vi "RTC DS1307 to LCD 16x2.vi"   [LabVIEW 2014]
doc: "This example shows how to read the current time from a DS1307 Real-Time Clock (RTC). This RTC is used on the Arduino Datalogger Shield, which also comes equipped with an SD card slot."
uses:
  <vilib>/Aledyne-TSXperts/Arduino Compatible Compiler for LabVIEW/Code Generator/Arduino APIs/I2C LCD/LiquidCrystal_I2C write String.vi
  <vilib>/Aledyne-TSXperts/Arduino Compatible Compiler for LabVIEW/Arduino Compatible Compiler for LabVIEW.lvlib
  QwaveSys_ESP8266/QwaveSys_ESP8266.lvlib
  QwaveSys_Interface/QwaveSys_Interface.lvlib
panel:
  # "These two wire for I2C (SDA,SCL) must be connected in order to use onboard RTC with Wemos D1 ESP8266 Board"
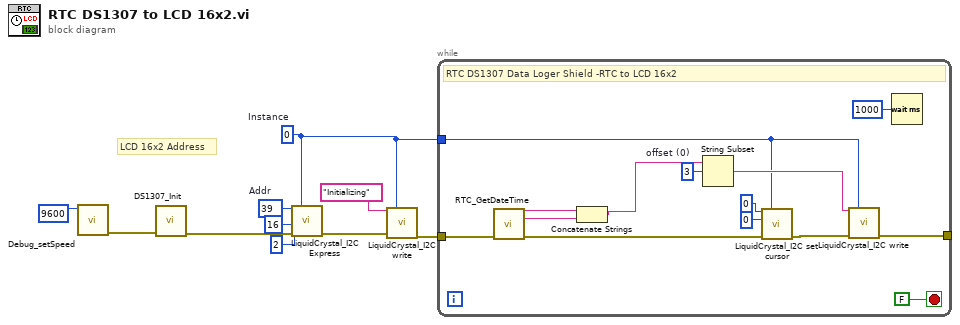
[diagram p0: block diagram]
diagram:
  w10 = u8 39  # Addr
  w4 = u8 0  # Instance
  # "LCD 16x2 Address"
  n1 = call "Debug_setSpeed.vi"("Speed"=u32 9600) -> ("error out"=w2:errorcluster)  [unwired: 10 in]
  n2 = call "DS1307_Init.vi"("error in (no error)"=w2) -> ("error out"=w1:errorcluster)  [unwired: 10 in]
  n3 = call <vilib>:"LiquidCrystal_I2C Express.vi"("Addr"=w10, "Instance"=w4, "Chars"=u16 16, "Lines"=u16 2, "error in (no error)"=w1) -> ("error out"=w7:errorcluster)  [unwired: 10 in]
  n4 = call-poly <vilib>:"LiquidCrystal_I2C write.vi"("Data"="Initializing", "Instance"=w4, "error in (no error)"=w7) -> ("error out"=w5:errorcluster)  [unwired: 12 in]
  n5 = while {
    tunnel: w5 -> [w15]
    tunnel: w4 -> [w19]
    tunnel: [w17] -> _
    stop <- FALSE stop-if-true
    w24 = 3  # offset (0)
    # "RTC DS1307 Data Loger Shield -RTC to LCD 16x2"
    n6 = call "RTC_GetDateTime.vi"("error in (no error)"=w15) -> ("error out"=w14:errorcluster, "time string"=w12:string, "date string"=w13:string)  [unwired: 8 in]
    n7 = Concatenate Strings(w13, w12) -> (w11:string)
    n8 = String Subset(string=w11, offset (0)=w24) -> (substring=w21:string)  [unwired: 1 in]
    n9 = call <vilib>:"LiquidCrystal_I2C set cursor.vi"("character"=u16 0, "Instance"=w19, "line"=u16 0, "error in (no error)"=w14) -> ("error out"=w20:errorcluster)  [unwired: 11 in]
    n10 = call-poly <vilib>:"LiquidCrystal_I2C write.vi"("Data"=w21, "Instance"=w19, "error in (no error)"=w20) -> ("error out"=w17:errorcluster)  [unwired: 12 in]
    n11 = Wait (ms)(milliseconds to wait=u32 1000) -> ()  [unwired: 1 out]
  }
